vi "ToPythonVersionString.vi"(11 "Enum":enum16{"2.7", "3.6", "3.10"}(ring)=enum."3.10") -> (3 "python version string":string)   [LabVIEW 2019]
doc: "Helper VI to convert from the Python version enum to a version string that is the input to the Open Python Session node."
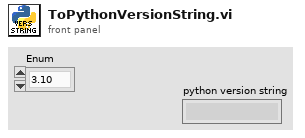
[diagram p1: front panel]
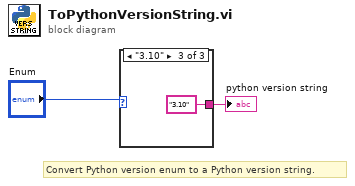
[diagram p0: block diagram]
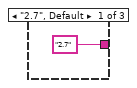
[diagram p2: hidden frame]
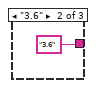
[diagram p3: hidden frame]
diagram:
  # "Convert Python version enum to a Python version string."
  n1 = case shown="\"3.10\"" "Enum" {
    tunnel: ["2.7" ("python version") "3.6" ("python version") "3.10" ("python version")] -> w2
    frame "2.7", Default {
    }
    frame "3.6" {
    }
    frame "3.10" {
    }
  }
  "python version string" <- w2
